vi "SourceCommand.vi"(2 "Parameter":i32, 3 "COM Port in":refnum<visa-resource-name>, 7 "Command":enum16{"S", "A"}(ring), 9 "entrée d'erreur":errorcluster caption="error in (no error)") -> (0 "COM Port out":refnum<visa-resource-name>, 1 "Error Code":i32, 6 "error out":errorcluster)   [LabVIEW 2009]
panel:
  out "Dialog":string
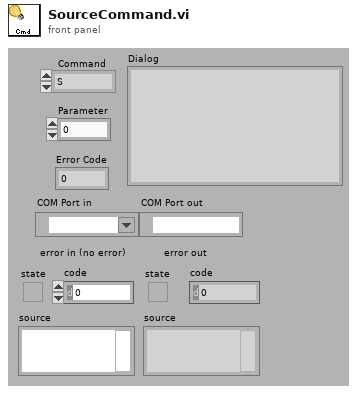
[diagram p1: front panel]
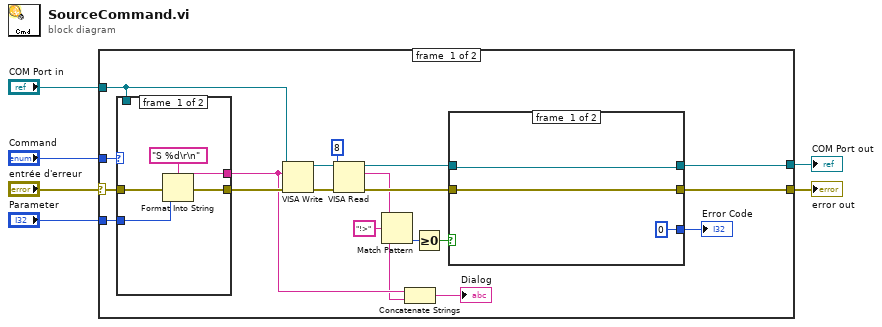
[diagram p0: block diagram]
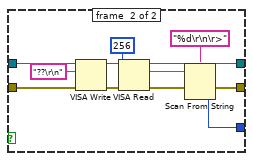
[diagram p2: hidden frame]
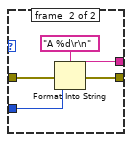
[diagram p3: hidden frame]
diagram:
  n1 = case shown="No Error" "entrée d'erreur" {
    selector: "entrée d'erreur" -> [w21 w52]
    tunnel: "Command" -> [w25 _]
    tunnel: "COM Port in" -> [w19 w51]
    tunnel: [w23 w52] -> w5
    tunnel: [w22 w51] -> w4
    tunnel: "Parameter" -> [w20 _]
    frame #0 {
      n2 = case shown="\"S\", Default" w25 {
        tunnel: w21 -> [w41 w46]
        tunnel: [w45 w50] -> w24
        tunnel: [w43 w48] -> w9
        tunnel: w20 -> [w42 w47]
        tunnel: w19 -> [_ _]
        frame #0 {
          n3 = Format Into String(format string="S %d\r\n" ("chaîne de format"), error in=w41, w42) -> (resulting string=w43:string, error out=w45:errorcluster)  [unwired: 1 in]
        }
        frame #1 {
          n4 = Format Into String(format string="A %d\r\n" ("chaîne de format"), error in=w46, w47) -> (resulting string=w48:string, error out=w50:errorcluster)  [unwired: 1 in]
        }
      }
      n5 = VISA Write(VISA resource name=w19, write buffer=w9, error in (no error)=w24) -> (VISA resource name out=w17:refnum<visa-resource-name>, error out=w18:errorcluster)  [unwired: 1 out]
      n6 = VISA Read(VISA resource name=w17, byte count=u32 8 ("nombre d'octets (0)"), error in (no error)=w18) -> (VISA resource name out=w15:refnum<visa-resource-name>, read buffer=w8:string, error out=w11:errorcluster)  [unwired: 1 out]
      n7 = Match Pattern(string=w8, regular expression="!>" ("expression")) -> (offset past match=w13:i32)  [unwired: 4 out]
      n8 = Concatenate Strings(w9, w8) -> (→"Dialog":string)
      n9 = Greater Or Equal To 0?(x=w13) -> (x >= 0?=w12:bool)
      n10 = case shown="True" w12 {
        tunnel: w11 -> [w28 w40]
        tunnel: w15 -> [w27 w39]
        tunnel: [w28 w31] -> w23
        tunnel: [w27 w34] -> w22
        tunnel: [0 w30] -> w10
        frame #0 {
        }
        frame #1 {
          n11 = VISA Write(VISA resource name=w39, write buffer="??\r\n" ("buffer à écrire"), error in (no error)=w40) -> (VISA resource name out=w35:refnum<visa-resource-name>, error out=w36:errorcluster)  [unwired: 1 out]
          n12 = VISA Read(VISA resource name=w35, byte count=u32 256 ("nombre d'octets (0)"), error in (no error)=w36) -> (VISA resource name out=w34:refnum<visa-resource-name>, read buffer=w29:string, error out=w32:errorcluster)  [unwired: 1 out]
          n13 = Scan From String(format string="%d\r\n\r>" ("chaîne de format"), input string=w29, error in=w32) -> (error out=w31:errorcluster, output 1=w30:i32)  [unwired: 1 in, 3 out]
        }
      }
      "Error Code" <- w10
    }
    frame #1 {
    }
  }
  "error out" <- w5
  "COM Port out" <- w4
